vi "Set Cell Type (Sheet).vi"(6 "Column":i32, 7 "Cell Type":T1=1 items=["Numeric"=0, "String"=1, "Formula"=2, "Blank"=3, "Boolean"=4, "Error"=5, "Unknown"=-1], 8 "error in (no error)":errorcluster, 9 "Row":i32, 10 "Sheet Reference":refnum<k24>) -> (0 "error out":errorcluster, 2 "Sheet Reference out":refnum<k24>)   [LabVIEW 2014]
uses:
  C:/PhaeronGit/LVNPOI/Resources/NPOI 2.1.1 dotnet2/NPOI.dll
  Resources/NPOI 2.1.1 dotnet2/NPOI.dll
  Typedefs/Cell Types.ctl
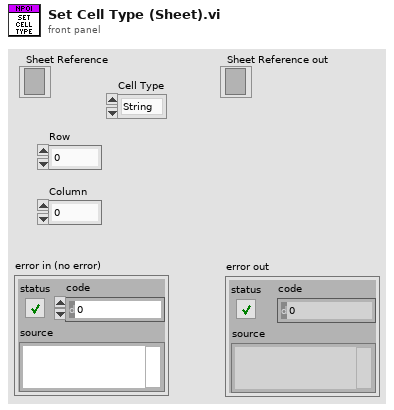
[diagram p1: front panel]
types:
  T1 = typedef "Cell Types.ctl" = i32
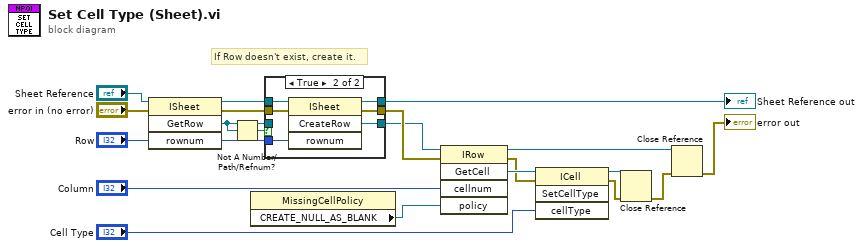
[diagram p0: block diagram]
diagram:
  # "If Row doesn't exist, create it."
  n1 = invoke class="ISheet" method="GetRow"(reference="Sheet Reference", error in="error in (no error)", "rownum"="Row") -> (reference out=w13:refnum<k24>, error out=w14:errorcluster, "GetRow"=w16:refnum<k24>)  [unwired: 1 in, 1 out]
  n2 = Not A Number/Path/Refnum?(number/path/refnum=w16) -> (NaN/Path/Refnum?=w15:bool)
  n3 = property class="MissingCellPolicy"() -> ("CREATE_NULL_AS_BLANK"=w6:refnum<k24>)  [unwired: 2 in, 2 out]
  n4 = case shown="True" w15 {
    tunnel: w13 -> [w23 w29]
    tunnel: w14 -> [w22 w28]
    tunnel: [w22 w27] -> w8
    tunnel: [w23 w26] -> w9
    tunnel: "Row" -> [_ w25]
    tunnel: [w21 w24] -> w7
    tunnel: w16 -> [w21 _]
    frame False {
    }
    frame True {
      n5 = invoke class="ISheet" method="CreateRow"(reference=w29, error in=w28, "rownum"=w25) -> (reference out=w26:refnum<k24>, error out=w27:errorcluster, "CreateRow"=w24:refnum<k24>)  [unwired: 1 in, 1 out]
    }
  }
  "Sheet Reference out" <- w9
  n6 = invoke class="IRow" method="GetCell"(reference=w7, error in=w8, "cellnum"="Column", "policy"=w6) -> (reference out=w20:refnum<k24>, error out=w1:errorcluster, "GetCell"=w2:refnum<k24>)  [unwired: 1 in, 2 out]
  n7 = invoke class="ICell" method="SetCellType"(reference=w2, error in=w1, "cellType"="Cell Type") -> (reference out=w4:refnum<k24>, error out=w5:errorcluster)  [unwired: 1 in, 2 out]
  n8 = Close Reference(reference=w4, error in (no error)=w5) -> (error out=w18:errorcluster)
  n9 = Close Reference(reference=w20, error in (no error)=w18) -> (error out=→"error out":errorcluster)
